vi "GetFloatValue.vi"(8 "error in (no error)":errorcluster caption="错误输入（无错误）", 10 "strValue":string, 11 "handle":u64) -> (0 "error out":errorcluster caption="错误输出", 1 "pFloatValue out":T1, 2 "function return":i32, 3 "handle out":u64)   [LabVIEW 2015, in "MvCameraControl.lvlib"]
doc: "MV_LV_API int __stdcall GetFloatValue( void* handle, const char* strValue, MVCC_FLOATVALUE *pFloatValue);"
uses:
  MvCameraControl.lvlib
  MvCameraControl.dll
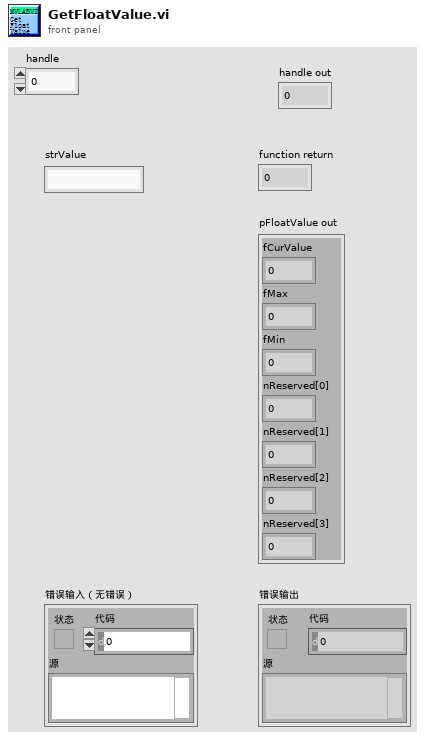
[diagram p1: front panel]
types:
  T1 = cluster{"fCurValue":sgl, "fMax":sgl, "fMin":sgl, "nReserved[0]":u32, "nReserved[1]":u32, "nReserved[2]":u32, "nReserved[3]":u32}
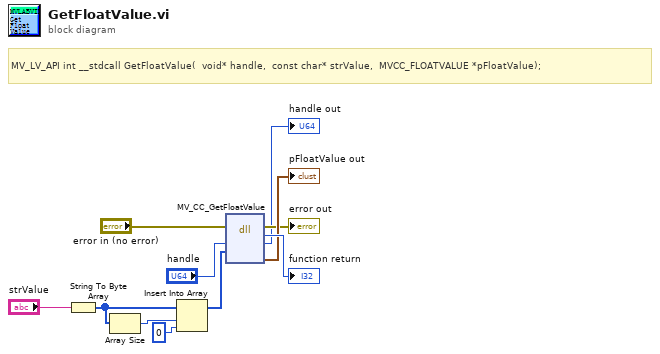
[diagram p0: block diagram]
diagram:
  # "MV_LV_API int __stdcall GetFloatValue(  void* handle,  const char* strValue,  MVCC_FLOATVALUE *pFloatValue);"
  n1 = String To Byte Array(string="strValue") -> (unsigned byte array=w7:u8[])
  n2 = Array Size(array=w7) -> (size(s)=w6:i32)
  n3 = Insert Into Array(array=w7, index=w6, new element=u8 0 ("新元素/子数组")) -> (w3:u8[])
  n4 = dll-call lib="MvCameraControl.dll" fn="MV_CC_GetFloatValue"(error in="error in (no error)", "handle"="handle", "strKey"=w3) -> (error out=→"error out":errorcluster, "返回类型"=→"function return":i32, "handle"=→"handle out":u64, "pFloatValue out"=→"pFloatValue out":T1)  [unwired: 4 in, 1 out]
